vi "provide_OME_data.vi"(6 "image ID":string, 8 "error in (no error)":errorcluster, 9 "structuredAttribute string in":string, 10 "OME element in":refnum<class "XMLElement.lvclass">, 11 "LightSourceMG090910LightEmittingDiode in":refnum<class "LightSourceMG090910LightEmittingDiode.lvclass">) -> (0 "error out":errorcluster, 1 "structuredAttribute string out":string, 2 "OME element out":refnum<class "XMLElement.lvclass">, 3 "LightSourceMG090910LightEmittingDiode out":refnum<class "LightSourceMG090910LightEmittingDiode.lvclass">)   [LabVIEW 2010, in "LightSourceMG090910LightEmittingDiode.lvclass"]
uses:
  LightSourceMG090910LightEmittingDiode.lvclass
  common/classes/XMLElement/XMLElement/XMLElement.lvclass
  GenericLightSource/GenericLightSource/GenericLightSource.lvclass
  Instrument/GenericInstrument/GenericInstrument/GenericInstrument.lvclass
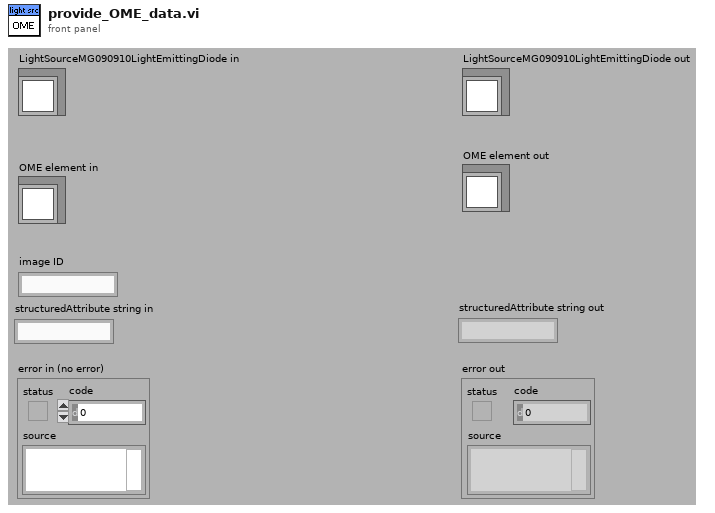
[diagram p1: front panel]
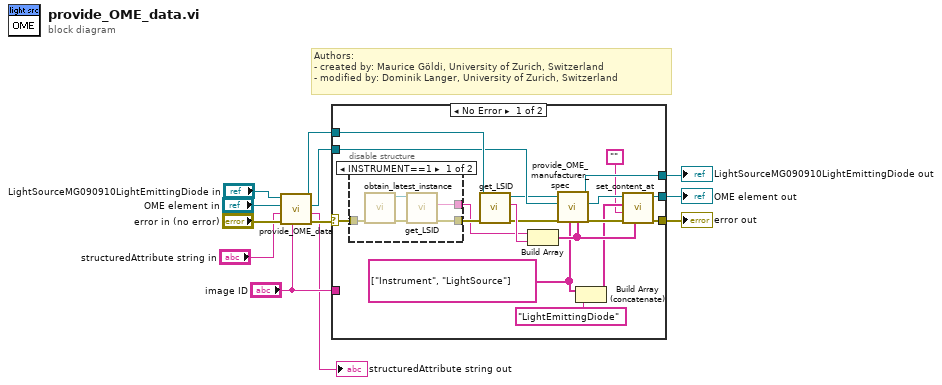
[diagram p0: block diagram]
diagram:
  # "Authors: \n- created by: Maurice Göldi, University of Zurich, Switzerland\n- modified by: Dominik Langer, University of Zurich, Switzerland"
  n1 = call-parent "provide_OME_data.vi"("image ID"="image ID", "error in (no error)"="error in (no error)", "structuredAttribute string in"="structuredAttribute string in", "OME element in"="OME element in", "GenericPlugin in"="LightSourceMG090910LightEmittingDiode in") -> ("error out"=w10:errorcluster, "structuredAttribute string out"=→"structuredAttribute string out":string, "OME element out"=w9:refnum<class "XMLElement.lvclass">, "GenericPlugin out"=w4:refnum<class "LightSourceMG090910LightEmittingDiode.lvclass">)  [unwired: 3 in]
  n2 = case shown="No Error" w10 {
    selector: w10 -> [w26 w37]
    tunnel: w9 -> [w15 w38]
    tunnel: w4 -> [w25 w39]
    tunnel: "image ID" -> [_ _]
    tunnel: [w20 w39] -> w7
    tunnel: [w30 w37] -> w8
    tunnel: [w24 w38] -> w5
    frame No Error {
      w18 = string[] ["Instrument", "LightSource"]
      n3 = disable-structure shown="INSTRUMENT==1" {
        disable-tunnel: w26 -> [w33 w36]
        disable-tunnel: [w32 w36] -> w28
        disable-tunnel: [w31 _] -> w27
        frame condition #0 {
          n4 = call "obtain_latest_instance.vi"("error in (no error)"=w33) -> ("error out"=w34:errorcluster, "microscope"=w35:refnum<class "GenericInstrument.lvclass">)  [unwired: 9 in]
          n5 = call-dynamic "get_LSID.vi"("error in (no error)"=w34, "GenericPlugin in"=w35) -> ("error out"=w32:errorcluster, "LSID (string)"=w31:string)  [unwired: 6 in, 2 out]
        }
        frame condition #1 (active) {
        }
      }
      n6 = call-dynamic "get_LSID.vi"("error in (no error)"=w28, "GenericPlugin in"=w25) -> ("error out"=w23:errorcluster, "LSID (string)"=w29:string, "GenericPlugin out"=w14:refnum<class "LightSourceMG090910LightEmittingDiode.lvclass">)  [unwired: 6 in, 1 out]
      n7 = Build Array(w27, w29) -> (w19:string[])
      n8 = call-dynamic "provide_OME_manufacturer_spec.vi"("id chain"=w19, "key chain"=w18, "error in (no error)"=w23, "XMLElement in"=w15, "GenericPlugin in"=w14) -> ("error out"=w22:errorcluster, "XMLElement out"=w21:refnum<class "XMLElement.lvclass">, "GenericPlugin out"=w20:refnum<class "LightSourceMG090910LightEmittingDiode.lvclass">)  [unwired: 4 in]
      n9 = Build Array (concatenate)(w18, "LightEmittingDiode") -> (w17:string[])
      n10 = call "set_content_at.vi"("id chain"=w19, "error in (no error)"=w22, "content"="", "key chain"=w17, "Element in"=w21) -> ("error out"=w30:errorcluster, "Element out"=w24:refnum<class "XMLElement.lvclass">)  [unwired: 5 in]
    }
    frame Error {
    }
  }
  "error out" <- w8
  "LightSourceMG090910LightEmittingDiode out" <- w7
  "OME element out" <- w5
